vi "User Interface.vi"(8 "error in (no error)":errorcluster, 11 "User Interface in":refnum<class "User Interface.lvclass">) -> (0 "error out":errorcluster, 3 "User Interface out":refnum<class "User Interface.lvclass">)   [LabVIEW 2023, in "UDPlog.lvlib" / "UDPlog Thread User Interface.lvclass"]
uses:
  UDPlog Thread User Interface.lvclass
  <vilib>/AddOns/VeriStand Custom Device Scripting APIs/Data Sharing Framework/DSF Core.lvlibp/Classes/User Interface/User Interface.lvclass
  Configurations/Thread/UDPlog Thread Configuration.lvclass
  Configurations/Thread/UDPlog Thread Configuration.lvclass/UDPlog Thread Configuration.ctl
  C:/Program Files/National Instruments/LabVIEW 2023/Vi.Lib/AddOns/VeriStand Custom Device Scripting APIs/Data Sharing Framework/DSF Core.lvlibp/Classes/Configuration/Configuration.lvclass
panel:
  in  "Local Address":string
  in  "Local Port":u16
  # "UDP Log UI"
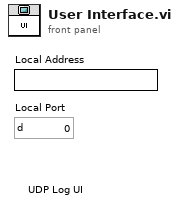
[diagram p1: front panel]
types:
  T1 = typedef "UDPlog.lvlib/UDPlog Thread Configuration.lvclass/Thread Settings.ctl" = cluster{"local port":u16, "local address":u32}
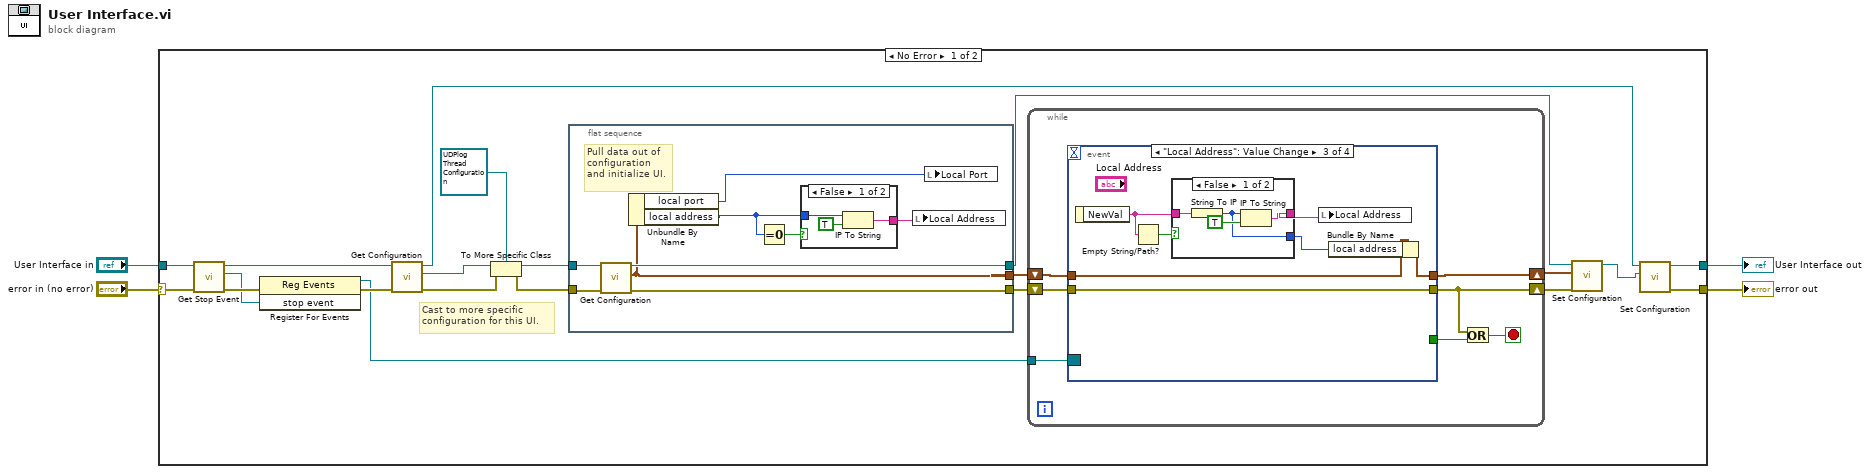
[diagram p0: block diagram]
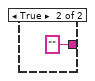
[diagram p2: hidden frame]
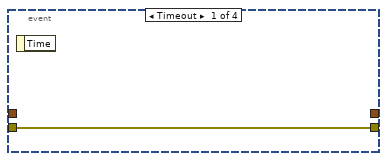
[diagram p3: hidden frame]
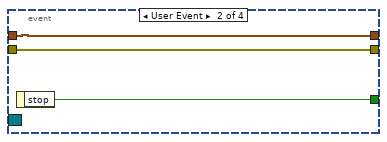
[diagram p4: hidden frame]
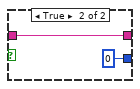
[diagram p5: hidden frame]
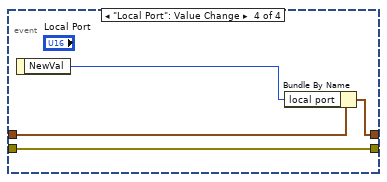
[diagram p6: hidden frame]
diagram:
  n1 = case shown="No Error" "error in (no error)" {
    selector: "error in (no error)" -> [w22 w68]
    tunnel: [w13 w68] -> w4
    tunnel: "User Interface in" -> [w21 w67]
    tunnel: [w12 w67] -> w1
    frame No Error {
      # "Cast to more specific configuration for this UI."
      n2 = call <vilib>:"Get Stop Event.vi"("error in (no error)"=w22, "User Interface in"=w21) -> ("error out"=w20:errorcluster, "stop event"=w19:refnum<user-event>, "User Interface out"=w18:refnum<class "User Interface.lvclass">)  [unwired: 7 in]
      n3 = register-events(error in=w20, w19) -> (reference out=w16:refnum<event-registration>, error out=w17:errorcluster)  [unwired: 1 in]
      n4 = call <vilib>:"Get Configuration.vi"("error in (no error)"=w17, "User Interface in"=w18) -> ("error out"=w15:errorcluster, "configuration"=w14:refnum<class "Configuration.lvclass">, "User Interface out"=w11:refnum<class "User Interface.lvclass">)  [unwired: 7 in]
      n5 = To More Specific Class(target class=refnum<class "UDPlog Thread Configuration.lvclass"> refnum ("UDPlog Thread Configuration in"), reference=w14, error in=w15) -> (specific class reference=w25:refnum<class "UDPlog Thread Configuration.lvclass">, error out=w23:errorcluster)
      n6 = flat-sequence {
        tunnel: [w32] -> w24
        tunnel: w23 -> [w33]
        tunnel: w25 -> [w34]
        tunnel: [w31] -> w5
        tunnel: [w28] -> w7
        frame #0 {
          # "Pull data out of configuration and initialize UI."
          n7 = call <vilib>:"Get Configuration.vi"("error in (no error)"=w33, "UDPlog Thread Configuration in"=w34) -> ("error out"=w32:errorcluster, "thread settings"=w28:T1, "UDPlog Thread Configuration out"=w31:refnum<class "UDPlog Thread Configuration.lvclass">)  [unwired: 7 in]
          n8 = Unbundle By Name(w28) -> ("local port"=w26:u16, "local address"=w27:u32)
          n9 = Equal To 0?(x=w27) -> (x = 0?=w30:bool)
          n10 = case shown="False" w30 {
            tunnel: [w37 "" ("name")] -> w29
            tunnel: w27 -> [w36 _]
            frame False {
              n11 = IP To String(1:TRUE ("dot notation? (F)"), 2:w36) -> (0:w37:string)
            }
            frame True {
            }
          }
          n12 = local write "Local Address"(w29) -> ()
          n13 = local write "Local Port"(w26) -> ()
        }
      }
      n14 = while {
        tunnel: w16 -> [w45]
        shift-right: [w43] -> w10
        shift-left: w24 -> [w44]
        shift-right: [w40] -> w6
        shift-left: w7 -> [w39]
        stop <- w42 stop-if-true
        n15 = event shown="[2] \"Local Address\": Value Change" {
          selector: w45 -> [_ _ _ _]
          dyn-events: _ -> [_ _ _ _]
          timeout: _ -> [_ _ _ _]
          tunnel: [_ w48 _ _] -> w41
          tunnel: w44 -> [w46 w49 w51 w66]
          tunnel: [w46 w49 w51 w66] -> w43
          tunnel: [_ w47 w54 w64] -> w40
          tunnel: w39 -> [_ w47 w55 w65]
          event Timeout {
            n16 = event-data() -> ()  [unwired: 1 in, 1 out]
          }
          event User Event {
            n17 = event-data() -> ("stop"=w48:bool)  [unwired: 1 in]
          }
          event "Local Address": Value Change {
            n18 = event-data() -> ("NewVal"=w56:string)  [unwired: 1 in]
            n19 = Empty String/Path?(string/path=w56) -> (empty?=w50:bool)
            n20 = case shown="False" w50 {
              tunnel: [w60 w61] -> w52
              tunnel: w56 -> [w59 w61]
              tunnel: [w57 u32 0] -> w53
              frame False {
                n21 = String To IP(1:w59) -> (0:w57:u32)
                n22 = IP To String(1:TRUE ("dot notation? (F)"), 2:w57) -> (0:w60:string)
              }
              frame True {
              }
            }
            n23 = local write "Local Address"(w52) -> ()
            n24 = Bundle By Name(cluster=w55, "local address"=w53) -> (w54:T1)
          }
          event "Local Port": Value Change {
            n25 = event-data() -> ("NewVal"=w63:u16)  [unwired: 1 in]
            n26 = Bundle By Name(cluster=w65, "local port"=w63) -> (w64:T1)
          }
        }
        n27 = Or(x=w43, y=w41) -> (x .or. y?=w42:bool)
      }
      n28 = call <vilib>:"Set Configuration.vi"("error in (no error)"=w10, "thread settings"=w6, "UDPlog Thread Configuration in"=w5) -> ("UDPlog Thread Configuration out"=w9:refnum<class "UDPlog Thread Configuration.lvclass">)  [unwired: 7 in, 1 out]
      n29 = call <vilib>:"Set Configuration.vi"("configuration"=w9, "User Interface in"=w11) -> ("error out"=w13:errorcluster, "User Interface out"=w12:refnum<class "User Interface.lvclass">)  [unwired: 8 in]
    }
    frame Error {
    }
  }
  "error out" <- w4
  "User Interface out" <- w1
